vi "Client.vi"() -> ()   [LabVIEW 2017]
panel:
  out "error out":errorcluster
  out "Waveform Chart":dbl[](graph)
  in  "# elements":i32
  in  "stop":bool
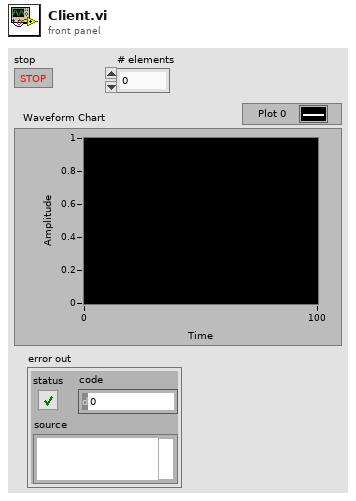
[diagram p1: front panel]
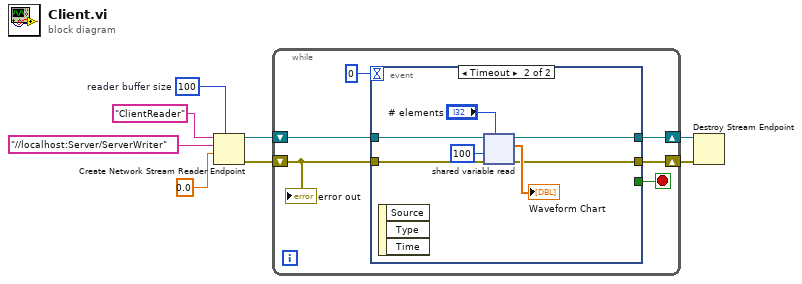
[diagram p0: block diagram]
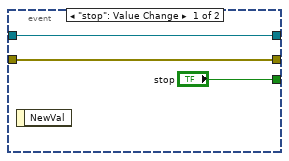
[diagram p2: hidden frame]
diagram:
  w5 = 100  # reader buffer size
  n1 = Create Network Stream Reader Endpoint(7:w5, 9:0.0, 10:"//localhost:Server/ServerWriter" ("writer url"), 11:"ClientReader" ("reader name")) -> (0:w3:errorcluster, 3:w4:refnum<k21>)  [unwired: 3 in]
  n2 = while {
    shift-right: [w10] -> w2
    shift-left: w3 -> [w11]
    shift-right: [w9] -> w1
    shift-left: w4 -> [w12]
    stop <- w14 stop-if-true
    n3 = event shown="[1] Timeout" {
      selector: _ -> [_ _]
      dyn-events: _ -> [_ _]
      timeout: 0 -> [_ _]
      tunnel: ["stop" _] -> w14
      tunnel: w12 -> [w15 w24]
      tunnel: w11 -> [w16 w23]
      tunnel: [w16 w20] -> w10
      tunnel: [w15 w19] -> w9
      event "stop": Value Change {
        n4 = event-data() -> ()  [unwired: 1 in, 1 out]
      }
      event Timeout {
        n5 = event-data() -> ()  [unwired: 1 in, 3 out]
        n6 = shared-variable-read(w24, w23, 100 ("timeout ms (-1)"), "# elements") -> (w19:refnum<k21>, w20:errorcluster, →"Waveform Chart":dbl[])  [unwired: 1 out]
      }
    }
    "error out" <- w11
  }
  n7 = Destroy Stream Endpoint(8:w2, 11:w1) -> ()  [unwired: 1 out]
